vi "Sort Types.vi"(11 "Types":T1[](array[typedef])) -> (3 "Sorted Types":T1[](array[typedef]))   [LabVIEW 2020, in "FlexBlock.xnode"]
uses:
  FlexBlock.xnode
  FlexBlocks/Terminal Direction.ctl
  FlexBlocks/FlexBlocks.lvlib
  FlexBlocks/Value Mode.ctl
  FlexBlocks/Terminal State.ctl
  FlexBlocks/Special Terminal.ctl
  FlexBlocks/Type Descriptor.ctl
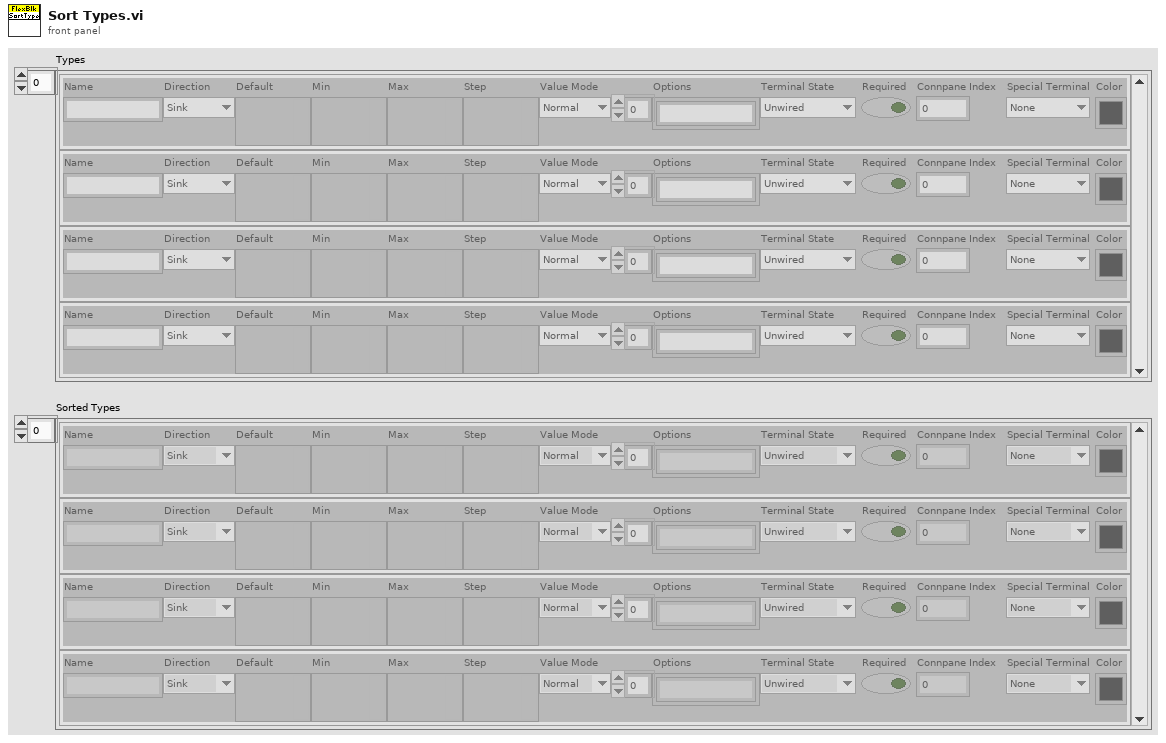
[diagram p1: front panel]
types:
  T1 = typedef "FlexBlocks.lvlib/Type Descriptor.ctl" = cluster{"Name":string, "Direction":T2, "Default":variant, "Min":variant, "Max":variant, "Step":variant, "Value Mode":T3, "Options":string[], "Terminal State":T4, "Required":bool, "Connpane Index":i32, "Special Terminal":T5, "Color":u32}
  T2 = typedef "FlexBlocks.lvlib/Terminal Direction.ctl" = enum16{"Sink", "Source"}
  T3 = typedef "FlexBlocks.lvlib/Value Mode.ctl" = enum16{"Normal", "Range", "Select"}
  T4 = typedef "FlexBlocks.lvlib/Terminal State.ctl" = enum16{"Unwired", "BadType", "BadRef", "Channel", "Value", "Control Ref"}
  T5 = typedef "FlexBlocks.lvlib/Special Terminal.ctl" = enum16{"None", "Action", "Init", "Tag", "State in", "State out", "Error"}
  T6 = cluster{i32, "Name":string, "Type Descriptor":T1}
  T7 = cluster{i32, "Name":string, "Type Descriptor":T1}[]
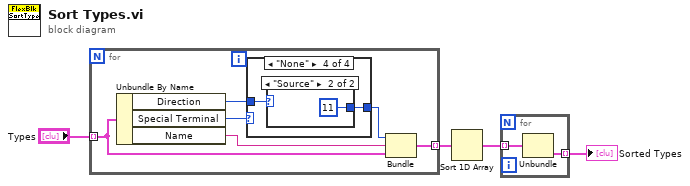
[diagram p0: block diagram]
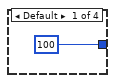
[diagram p2: hidden frame]
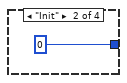
[diagram p3: hidden frame]
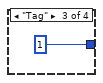
[diagram p4: hidden frame]
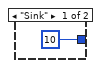
[diagram p5: hidden frame]
diagram:
  n1 = for {
    tunnel: "Types" -> [w9] mode=indexing
    tunnel: [w5] -> w3 mode=indexing
    n2 = Unbundle By Name(w9) -> ("Direction"=w6:T2, "Special Terminal"=w8:T5, "Name"=w10:string)
    n3 = case shown="\"None\"" w8 {
      tunnel: [100 0 1 w14] -> w7
      tunnel: w6 -> [_ _ _ w15]
      frame Default {
      }
      frame "Init" {
      }
      frame "Tag" {
      }
      frame "None" {
        n4 = case shown="\"Source\"" w15 {
          tunnel: [10 11] -> w14
          frame "Sink" {
          }
          frame "Source" {
          }
        }
      }
    }
    n5 = Bundle(w7, "Name"=w10, "Type Descriptor"=w9) -> (w5:T6)  [unwired: 1 in]
  }
  n6 = Sort 1D Array(array=w3) -> (sorted array=w2:T7)
  n7 = for {
    tunnel: w2 -> [w19] mode=indexing
    tunnel: [w18] -> w1 mode=indexing
    n8 = Unbundle(w19) -> ("Type Descriptor"=w18:T1)  [unwired: 2 out]
  }
  "Sorted Types" <- w1
